vi "Zählerwert_lesen.vi"(11 "Band/Station Index":T1) -> (0 "Zählerwert 3":u16, 1 "Zählerwert 2":u16, 3 "Zählerwert 1":u16)   [LabVIEW 2013, in "cRIO_FPGA_COMMUNICATION.lvlib"]
uses:
  cRIO_FPGA_COMMUNICATION.lvlib
  TYPES/TYPE Station Index.ctl
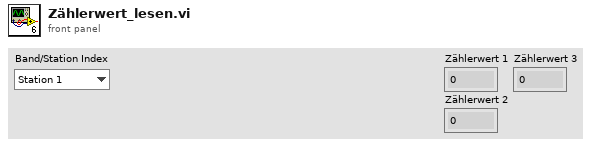
[diagram p1: front panel]
types:
  T1 = typedef "cRIO_FPGA_COMMUNICATION.lvlib/TYPE Station Index.ctl" = enum16{"Station 1", "Station 2", "Station 3", "Station 4", "Station 5", "Station 6", "Station 7", "Station 8", "Station 9", "Station 10", "Station 11", "Station 12", "Station 13", "Station 14", "Station 15", "Station 16", "Station 17", "Station 18", "Station 19", "Station 20"}
  T2 = enum16{"Init", "Zählerwert updaten", "Zählerwert lesen"}
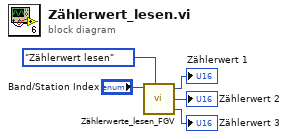
[diagram p0: block diagram]
diagram:
  n1 = call "Zählerwerte_lesen_FGV.vi"("Band/Station Index"="Band/Station Index", "Modus"=T2."Zählerwert lesen") -> ("Zählerwert 1"=→"Zählerwert 1":u16, "Zählerwert 2"=→"Zählerwert 2":u16, "Zählerwert 3"=→"Zählerwert 3":u16)  [unwired: 3 in]
